vi "Initialize.vi"(6 "Default return":variant, 7 "reader buffer size":i32=4096, 8 "error in (no error)":errorcluster, 9 "connection timeout":i32=-1, 10 "writer url":string, 11 "reader name":string) -> (0 "error out":errorcluster, 1 "Initialized?":bool, 3 "NetworkStreamWriter out":refnum<class "NetworkStreamReader.lvclass">)   [LabVIEW 2011, in "NetworkStreamReader.lvclass"]
doc: "This VI returns an instance of the NetworkStreamReader class. A NetworkStreamReader attempts to open a network stream with a writer endpoint. As with network streams, the writer url on the reader or the reader url on the writer must be given before the connection can be made. Note that until a connection is made, this VI will not return. It will, however, stop on a commanded e-stop from the top-level VI. This VI also launches a reader daemon which constantly adds information passed across the stream to an internal queue accessed by the Read method."
uses:
  NetworkStreamReader.lvclass
  Shared/message.ctl
  Shared/messageQueue.ctl
  NetworkStreamReader.lvclass/NetworkStreamReader.ctl
  ReaderDaemon.vi
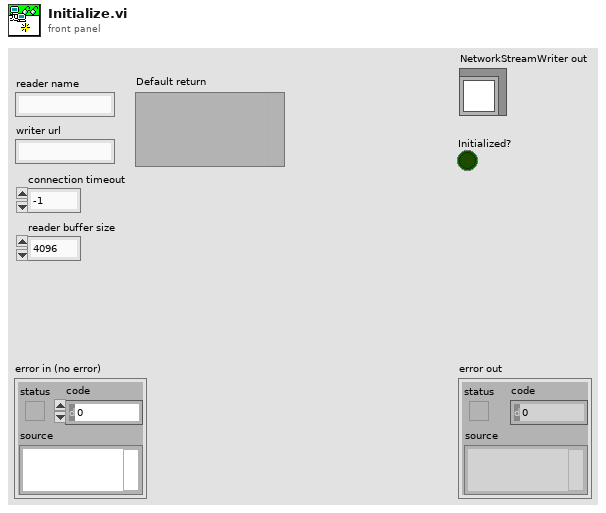
[diagram p1: front panel]
types:
  T1 = typedef "message.ctl" = cluster{"Data":variant, "Time since start (s)":dbl}
  T2 = typedef "messageQueue.ctl" = refnum<queue>
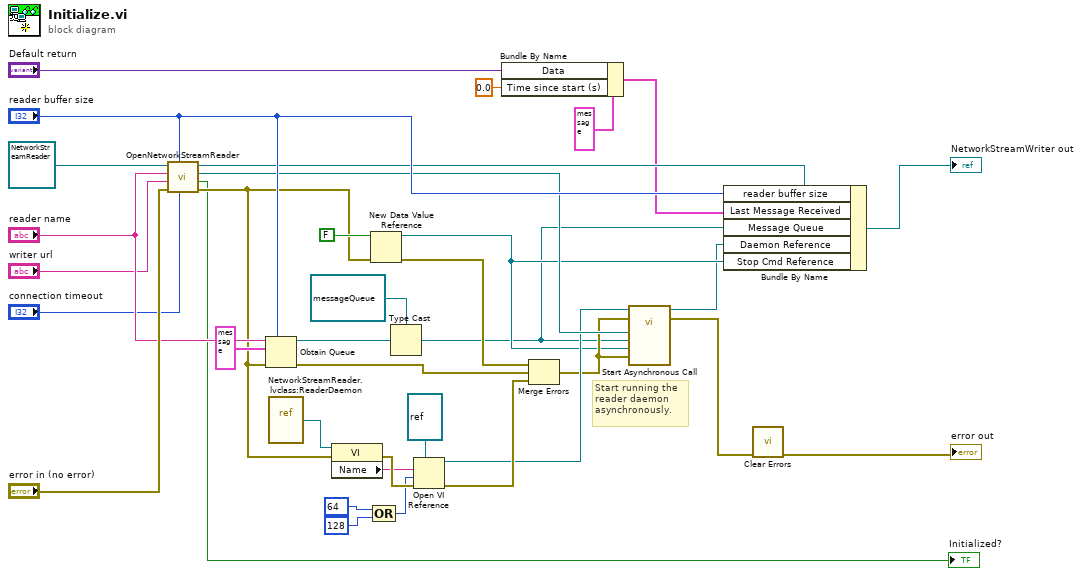
[diagram p0: block diagram]
diagram:
  # "Start running the \nreader daemon\nasynchronously."
  n1 = call "OpenNetworkStreamReader.vi"("connection timeout"="connection timeout", "reader buffer size"="reader buffer size", "error in (no error)"="error in (no error)", "writer url"="writer url", "reader name"="reader name", "NetworkStreamReader in"=refnum<class "NetworkStreamReader.lvclass"> refnum ("NetworkStreamWriter in")) -> ("error out"=w4:errorcluster, "Initialized?"=→"Initialized?":bool, "Reader Endpoint"=w21:refnum<k21>, "NetworkStreamReader out"=w8:refnum<class "NetworkStreamReader.lvclass">)  [unwired: 2 in]
  n2 = Obtain Queue(max queue size (-1, unlimited)="reader buffer size", name (unnamed)="reader name", element data type=T1 {"Data"=variant, "Time since start (s)"=0.0}, error in (no error)=w4) -> (queue out=w11:refnum<queue>, error out=w27:errorcluster)  [unwired: 1 in, 1 out]
  n3 = vi-ref "NetworkStreamReader.lvclass:ReaderDaemon.vi"() -> (w23:refnum<vi>)
  n4 = property class="VI"(reference=w23, error in=w4) -> (error out=w26:errorcluster, "Name"=w24:string)  [unwired: 1 out]
  n5 = New Data Value Reference(data value=FALSE, error in=w4) -> (data value reference=w13:refnum<data-value>, error out=w15:errorcluster)
  n6 = Compound Arithmetic op=OR(64 ("options"), 128 ("options")) -> (w17:i32)
  n7 = Type Cast(type=T2 refnum ("Variant Queue"), x=w11) -> (*(type *) &x=w9:T2)
  n8 = Open VI Reference(type specifier VI Refnum (for type only)=refnum<vi> refnum, vi path=w24, options=w17, error in (no error)=w26) -> (vi reference=w20:refnum<vi>, error out=w22:errorcluster)  [unwired: 2 in]
  n9 = Bundle By Name(cluster=T1 {"Data"=variant, "Time since start (s)"=0.0} ("Last Message Received"), "Data"="Default return", "Time since start (s)"=0.0) -> (w5:T1)
  n10 = Merge Errors(w15, w27, w22) -> (w16:errorcluster)
  n11 = call-by-ref "Start Asynchronous Call"(reference=w20, error in=w16, 8:"error in (no error)"=w16, "Stop command reference"=w13, "Variant Queue"=w9, "Reader Endpoint"=w21) -> (reference out=w12:refnum<vi>, error out=w2:errorcluster)  [unwired: 8 in]
  n12 = Bundle By Name(cluster=w8, "reader buffer size"="reader buffer size", "Last Message Received"=w5, "Message Queue"=w9, "Daemon Reference"=w12, "Stop Cmd Reference"=w13) -> (→"NetworkStreamWriter out":refnum<class "NetworkStreamReader.lvclass">)
  n13 = call <vilib>:"Clear Errors.vi"("error in (no error)"=w2) -> ("error out"=→"error out":errorcluster)  [unwired: 6 in]
